vi "Data_aq.vi"() -> ()   [LabVIEW 2016]
doc: "Use this template to measure or generate signals using the DAQ Assistant Express VI and NI-DAQmx. Double click the DAQ Assistant Express VI to launch a configuration wizard which steps you through configuring a measurement or generation.\n\nNote: You must have an NI-DAQmx compatible device installed to use this Express VI. Refer to the DAQ Quick Start Guide for NI-DAQ 7.0 for a list of compatible devices."
uses:
  <vilib>/Platform/TimedLoop/XDataNode/timing_clust.ctl
  <vilib>/Platform/TimedLoop/XDataNode/nitl_modes.ctl
  <vilib>/Platform/TimedLoop/XDataNode/wakeup.ctl
  <vilib>/Utility/file.llb/Write Delimited Spreadsheet (string).vi
  <vilib>/Platform/TimedLoop/XDataNode/loadnilvce.vi
  <vilib>/Utility/file.llb/Write Delimited Spreadsheet (DBL).vi
  <vilib>/express/express shared/transition.llb/Dynamic To Waveform Array.vi
  <vilib>/express/express signal manip/GetorSetDDTAttributes/Set DDT Attributes/SetT0.vi
  <vilib>/express/express shared/transition.llb/Waveform Array To Dynamic.vi
  <vilib>/Platform/TimedLoop/XDataNode/XDataNode.xnode
  <vilib>/express/express signal manip/GetorSetDDTAttributes/Set DDT Attributes/Set DDT Properties.xnode
  <vilib>/Platform/TimedLoop/XDataNode/XDNodeRunTimeDep.lvlib
  <resource>/objmgr/ni.var.rc
panel:
  out "NH4 Probe":refnum<k21>="ni.var.io://localhost/Mod6/AI0"
  out "Na Probe":refnum<k21>="ni.var.io://localhost/Mod6/AI1"
  out "new file path (Not A Path if cancelled)":path
  in  "File Name:":string
  out "Saving?":bool
  out "Headers":string[](array[string])
  out "error out":errorcluster
  out "Na Live":dbl format="%#_4g"
  out "String 6":string="Na"
  in  "error in":errorcluster
  out "NH4 Live":dbl format="%#_4g"
  out "All data":dbl[][](array[numeric]) format="%#3.4f"
  out "current sample":dbl format="%#_3g"
  out "Time":string="K"
  out "Date":string="K"
  out "iter number":i32
  out "String 2":string="NH4"
  in  "stop":bool
  # "Live"
  # "Last 50"
  # "Last 100"
  # "All"
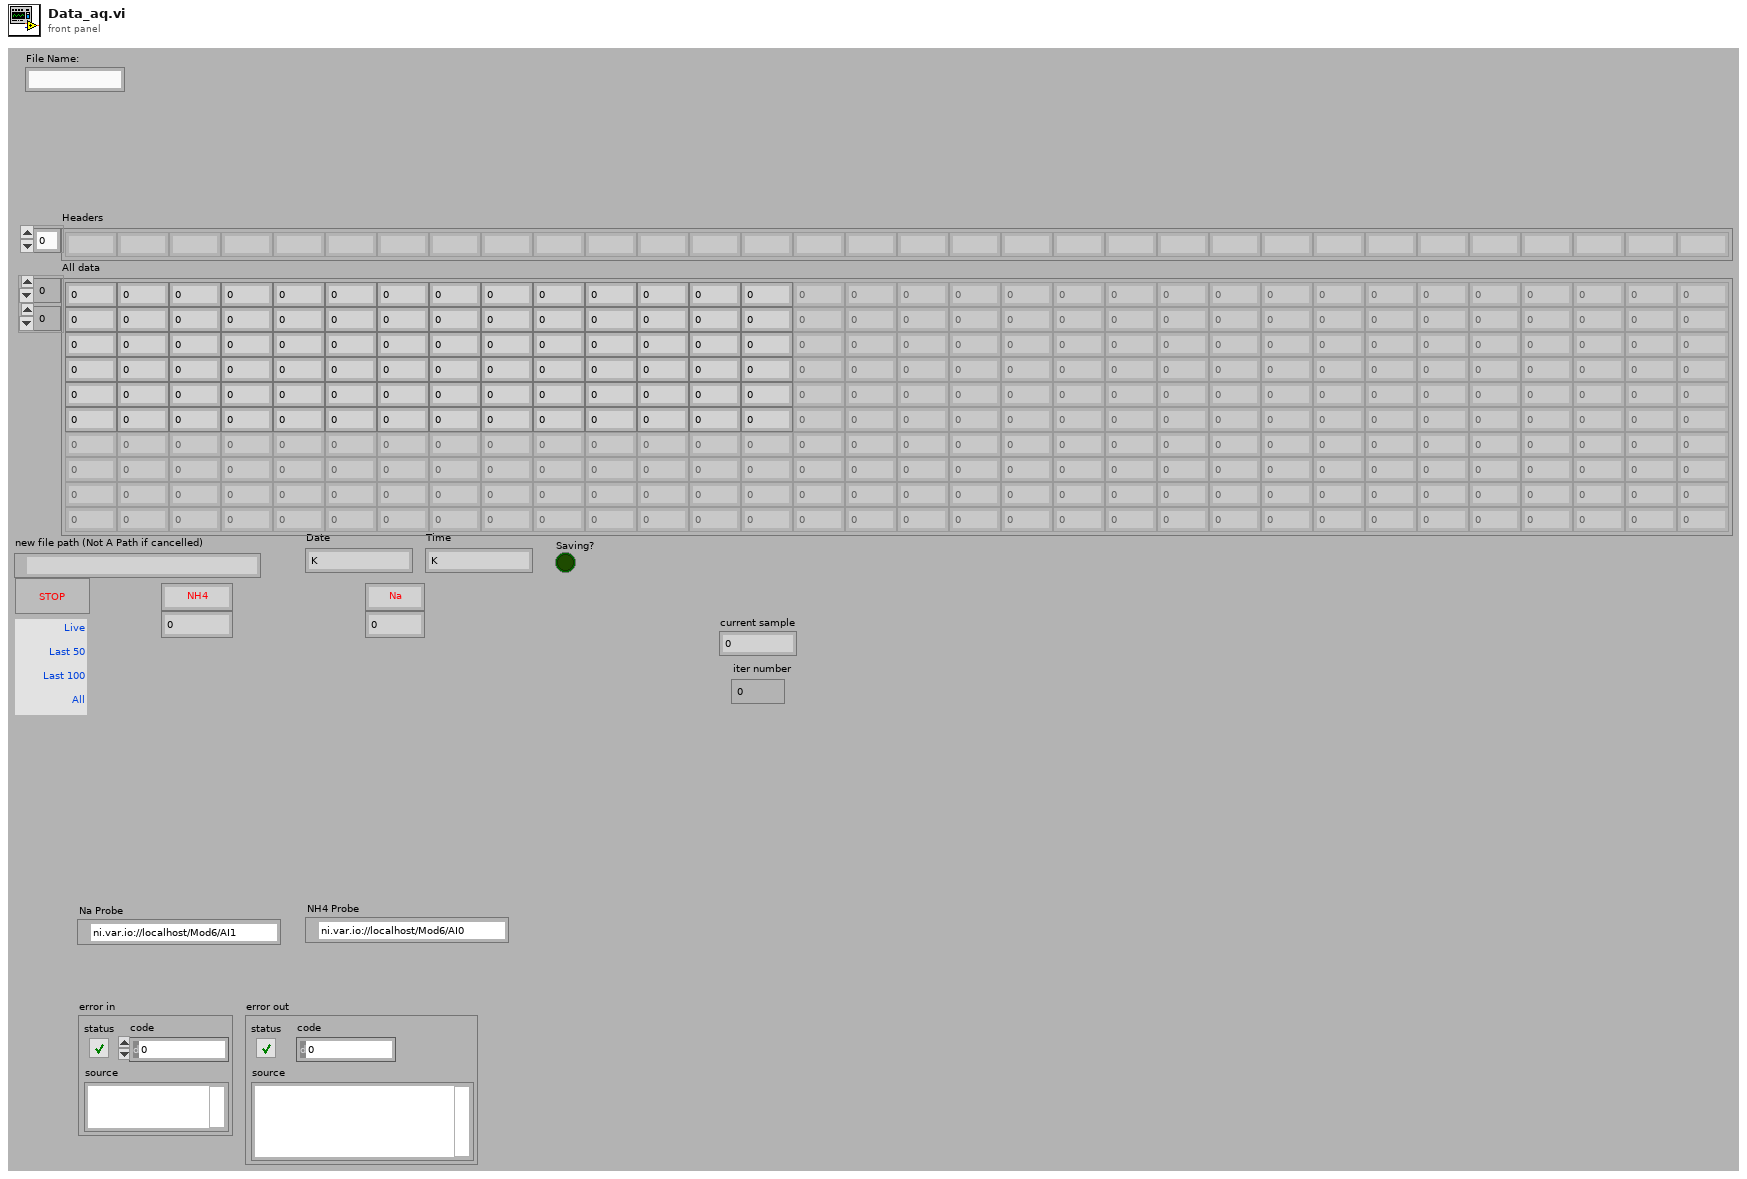
[diagram p1: front panel]
types:
  T1 = enum16{"open", "replace", "create", "open or create", "replace or create", "replace or create with confirmation"}
  T2 = typedef "XDNodeRunTimeDep.lvlib/timing_clust.ctl" = cluster{"Expected End [f-1]":u64, "Actual End [f-1]":u64, "Finished Late? [f-1]":bool, "Expected End [i-1]":u64, "Actual End [i-1]":u64, "Finished Late? [i-1]":bool, "Expected Start [i]":u64, "Actual Start [i]":u64, "Expected Start [f]":u64, "Actual Start [f]":u64, "Source Name":string, "Structure Name":string, "Period":i64, "Deadline":i64, "Offset":i64, "Start":i64, "Priority":i32, "Timeout":i32, "Mode":T3, "Wakeup Reason":T4, "Error":errorcluster, "Source Type":string, "Secondary Source Type":string, "Global End Time":u64, "Global Start Time":u64, "Frame Duration":u64, "Iteration Duration":u64, "Assigned CPU":i32, "I/O Scan Engine Mode":u32}
  T3 = typedef "XDNodeRunTimeDep.lvlib/nitl_modes.ctl" = enum32{"No Change", "Process missed periods, maintain original phase", "Discard missed periods, maintain original phase", "Process missed periods, ignore original phase", "Discard missed periods, ignore original phase"}
  T4 = typedef "XDNodeRunTimeDep.lvlib/wakeup.ctl" = enum32{"Normal", "Aborted", "Asynchronous wakeup", "Timing source error", "Timed loop error", "Timeout"}
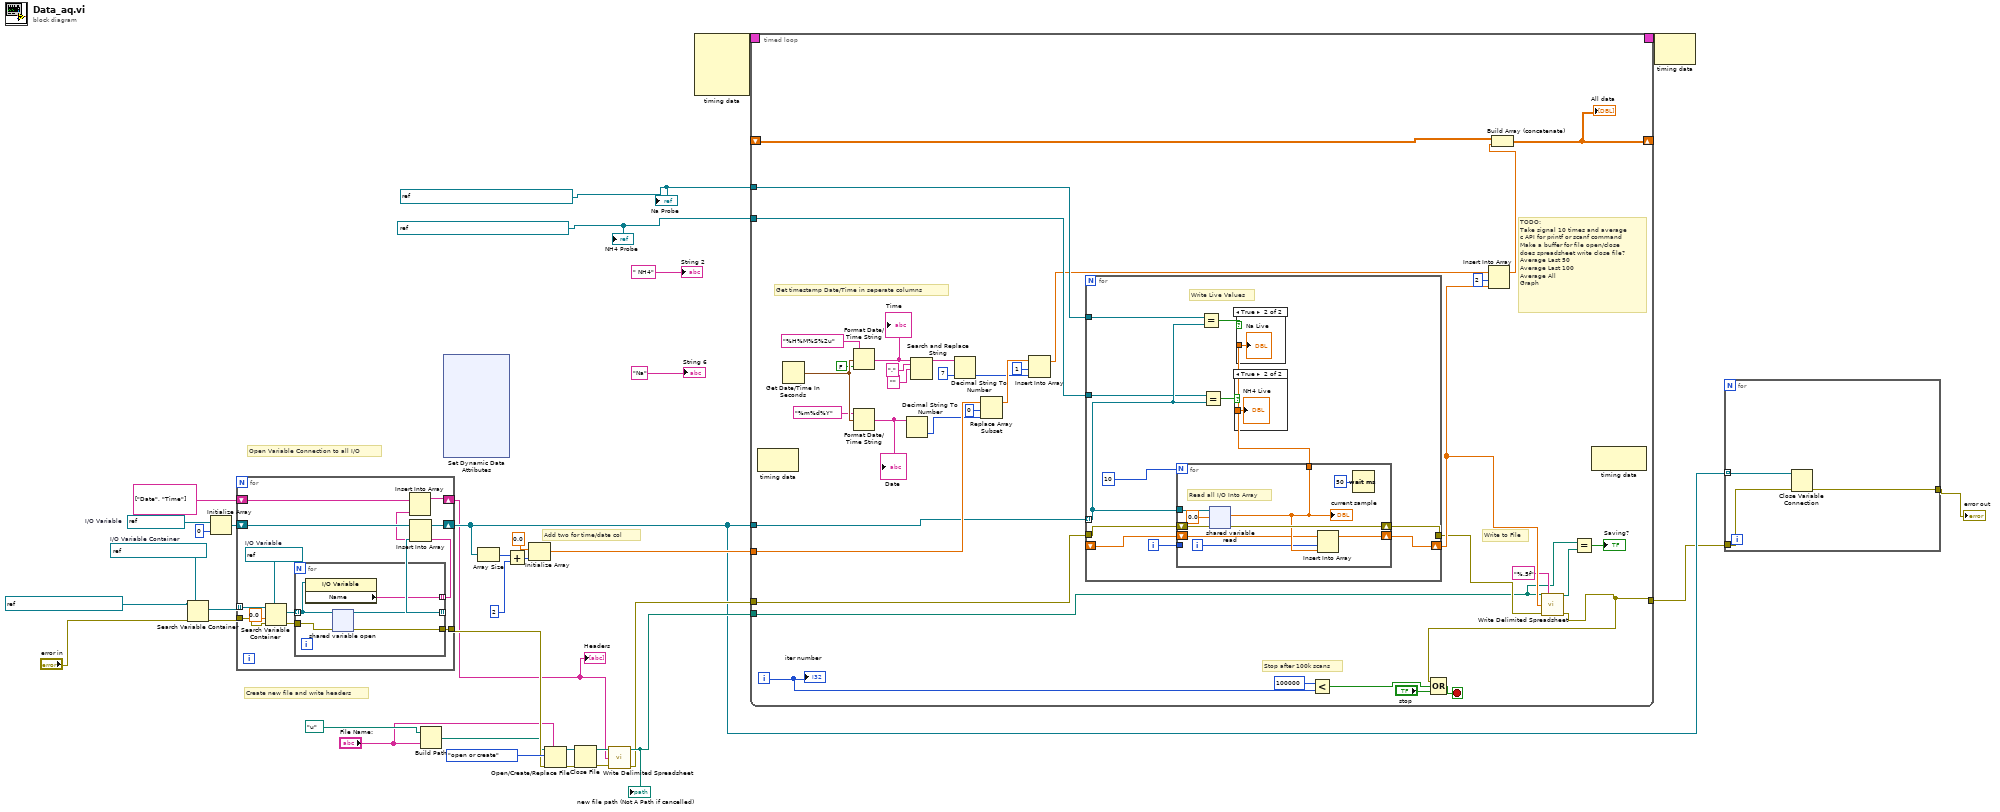
[diagram p0: block diagram]
diagram:
  w2 = refnum<k21> "ni.var.io://localhost/Mod6/AI1" ("Variable Name Control/Indicator")
  w1 = refnum<k21> "ni.var.io://localhost/Mod6/AI0" ("Variable Name Control/Indicator")
  w30 = refnum<k21> refnum  # I/O Variable
  w33 = refnum<k21> refnum  # I/O Variable Container
  # "Create new file and write headers"
  # "Add two for time/date col"
  # "Open Variable Connection to all I/O"
  n1 = Search Variable Container(7:w33, 8:"error in", 11:refnum<k21> "ni.var.io://crio1-winklerlab" ("Variable Name Control/Indicator")) -> (0:w32:errorcluster, 2:w34:refnum<k21>[])  [unwired: 3 in, 1 out]
  n2 = Initialize Array(w30, 0 ("dimension size")) -> (w31:refnum<k21>[])
  n3 = for {
    tunnel: w34 -> [w48] mode=indexing
    tunnel: w32 -> [w44]
    shift-right: [w40] -> w10
    shift-left: w31 -> [w41]
    tunnel: [w39] -> w12
    shift-right: [w37] -> w6
    shift-left: string[] ["Date", "Time"] -> [w38]
    w47 = refnum<k21> refnum  # I/O Variable
    n4 = Search Variable Container(7:w47, 8:w44, 9:0.0, 11:w48) -> (0:w43:errorcluster, 2:w46:refnum<k21>[])  [unwired: 2 in, 1 out]
    n5 = for {
      tunnel: w46 -> [w50] mode=indexing
      tunnel: w43 -> [w53]
      tunnel: [w52] -> w42 mode=indexing
      tunnel: [w51] -> w39
      tunnel: [w49] -> w36 mode=indexing
      n6 = property class="I/O Variable"(reference=w50) -> ("Name"=w49:string)  [unwired: 1 in, 2 out]
      n7 = shared-variable-open(w50, w53) -> (w52:refnum<k21>, w51:errorcluster)  [unwired: 1 in]
    }
    n8 = Insert Into Array(array=w38, new element=w36) -> (w37:string[])  [unwired: 1 in]
    n9 = Insert Into Array(array=w41, new element=w42) -> (w40:refnum<k21>[])  [unwired: 1 in]
  }
  "Headers" <- w6
  n10 = Build Path(base path=path "u:/" ("Save to:"), name or relative path="File Name:") -> (appended path=w4:path)
  n11 = xnode "Set Dynamic Data Attributes"() -> ()  [unwired: 4 in, 2 out]
  n12 = Array Size(array=w10) -> (size(s)=w24:i32)
  n13 = Add(x=w24, y=2) -> (x+y=w22:i32)
  n14 = Initialize Array(0.0, w22) -> (w25:dbl[])
  n15 = Open/Create/Replace File(file path (use dialog)=w4, error in=w12, prompt="File Name:", operation (0:open)=T1."open or create") -> (refnum out=w17:refnum<file>, error out=w18:errorcluster)  [unwired: 2 in, 1 out]
  n16 = Close File(refnum=w17, error in=w18) -> (path=w16:path, error out=w13:errorcluster)
  n17 = call-poly <vilib>:"Write Delimited Spreadsheet.vi"("file path (dialog if empty)"=w16, "1D data"=w6, "error in (no error)"=w13) -> ("new file path (Not A Path if cancelled)"=w15:path, "error out"=w11:errorcluster)  [unwired: 11 in]
  "new file path (Not A Path if cancelled)" <- w15
  n18 = node-c288() -> (w28:T2)  [unwired: 4 in]
  n19 = timed-loop {
    timing: w28 -> [_]
    timing-out: [_] -> w27
    tunnel: w10 -> [w72]
    tunnel: w25 -> [w80]
    tunnel: w11 -> [w90]
    tunnel: w15 -> [w56]
    tunnel: w2 -> [w73]
    tunnel: w1 -> [w74]
    shift-right: [w69] -> _
    shift-left: _ -> [w70]
    tunnel: [w54] -> w9
    i -> [w71]
    stop <- w76 stop-if-true
    # "TODO: \nTake signal 10 times and average\nc API for printf or scanf command\nMake a buffer for file open/close \ndoes spreadsheet write close file?\nAverage Last 50\nAverage Last 100\nAverage All\nGraph"
    # "Stop after 100k scans"
    # "Write to File"
    # "Get timestamp Date/Time in seperate columns"
    n20 = node-c288() -> ()  [unwired: 1 in, 1 out]
    n21 = Get Date/Time In Seconds() -> (seconds since 1Jan1904=w88:timestamp)
    n22 = Format Date/Time String(time format string (%c)="%H%M%S%2u", seconds (now)=w88, UTC format=FALSE) -> (date/time string=w84:string)
    "Time" <- w84
    n23 = Format Date/Time String(time format string (%c)="%m%d%Y", seconds (now)=w88) -> (date/time string=w67:string)  [unwired: 1 in]
    "Date" <- w67
    n24 = Decimal String To Number(string=w67) -> (number=w66:i32)  [unwired: 2 in, 1 out]
    n25 = Search and Replace String(input string=w84, search string=".", replace string="") -> (result string=w83:string)  [unwired: 5 in, 3 out]
    n26 = Decimal String To Number(string=w83, default (0L)=7) -> (number=w65:i32)  [unwired: 1 in, 1 out]
    n27 = Replace Array Subset(array=w80, new element=w66, index=0) -> (w79:dbl[])
    n28 = Insert Into Array(array=w79, index=1, new element=w65) -> (w64:dbl[])
    n29 = for {
      tunnel: w72 -> [w100] mode=indexing
      tunnel: w90 -> [w102]
      shift-right: [w91] -> w61
      shift-left: _ -> [w92]
      tunnel: [w101] -> w59
      tunnel: w74 -> [w99]
      tunnel: w73 -> [w97]
      i -> [w93]
      # "Write Live Values"
      n30 = for {
        N: 10 -> [_]
        tunnel: w100 -> [w108]
        tunnel: [w107] -> w98
        tunnel: w93 -> [_]
        shift-right: [w109] -> w101
        shift-left: w102 -> [w111]
        shift-right: [w103] -> w91
        shift-left: w92 -> [w105]
        i -> [w104]
        # "Read all I/O Into Array"
        n31 = shared-variable-read(w108, w111, 0.0) -> (w109:errorcluster, w107:dbl)  [unwired: 2 out]
        "current sample" <- w107
        n32 = Insert Into Array(array=w105, index=w104, new element=w107) -> (w103:dbl[])
        n33 = Wait (ms)(milliseconds to wait=u32 50) -> ()  [unwired: 1 out]
      }
      n34 = Equal?(x=w97, y=w100) -> (x = y?=w95:bool)
      n35 = Equal?(x=w99, y=w100) -> (x = y?=w96:bool)
      n36 = case shown="True" w96 {
        tunnel: w98 -> [_ w113]
        frame False {
        }
        frame True {
          "NH4 Live" <- w113
        }
      }
      n37 = case shown="True" w95 {
        tunnel: w98 -> [_ w112]
        frame False {
        }
        frame True {
          "Na Live" <- w112
        }
      }
    }
    n38 = Less?(x=100000, y=w71) -> (x < y?=w75:bool)
    n39 = Insert Into Array(array=w64, index=2, new element=w61) -> (w62:dbl[])
    n40 = Build Array (concatenate)(w70, w62) -> (w69:dbl[][])
    "All data" <- w69
    n41 = call-poly <vilib>:"Write Delimited Spreadsheet.vi"("file path (dialog if empty)"=w56, "format (%.3f)"="%.5f", "1D data"=w61, "error in (no error)"=w59) -> ("new file path (Not A Path if cancelled)"=w57:path, "error out"=w54:errorcluster)  [unwired: 10 in]
    n42 = Compound Arithmetic op=OR(w54, w75, "stop") -> (w76:bool)
    n43 = Equal?(x=w56, y=w57) -> (x = y?=→"Saving?":bool)
    n44 = node-c288() -> ()  [unwired: 1 in, 1 out]
    "iter number" <- w71
  }
  n45 = node-c288(w27) -> ()  [unwired: 1 out]
  n46 = for {
    tunnel: w10 -> [w118] mode=indexing
    tunnel: w9 -> [w117]
    tunnel: [w116] -> w8
    n47 = Close Variable Connection(8:w117, 11:w118) -> (0:w116:errorcluster)
  }
  "error out" <- w8
  "String 2" <- " NH4"
  "String 6" <- "Na"
  "Na Probe" <- w2
  "NH4 Probe" <- w1
